vi "Calculo principal.vi"(8 "error in":errorcluster, 11 "Dados SP":T2={"Condutor"={"Pc (N/m)"=0.0, "Mod.Young (N/m²)"=0.0, "Dil.Term.c (m/°C)"=0.0, "Área  (m²)"=0.0, "Tração EDS (N)"=0.0, "Tração Torig(N)"=0.0, "Tração Talta (N)"=0.0}, "Suporte"={"Ps (N/m)"=0.0, "Es (N/m²)"=0.0, "DTc (1/°C)"=0.0, "Área sup (m²)"=0.0, "Tração EDS sup (N)"=0.0, "Tração AT sup (N)"=0.0, "Flecha sup AT (m)"=0.0}, "Projeto"={"Temp. EDS (°C)"=0.0, "Lim.original (°C)"=0.0, "Lim.extend. (°C)"=0.0, "N. cabo/fase"=1.0}, "Vetor de dados"={"Coor.X.esp"=[], "Coor.Y.Esp."=[], "Sub.vao X"=[], "Sub.vao Y"=[], "CoordY.sup"=[], "CoordX.sup"=[]}, "Subvão"={"N. Esp."=0.0, "F.lim (m)"=0.0, "Ext.calc"=0.0, "Ext.definido"=0.0, "Comp.cabo"=0.0, "Ext.55%"=0.0, "Tração sub\nAT (N)"=0.0, "Ext.sel."=0.0, "Flecha lim.\ncalc (m)"=0.0}, "Vão"={"Extensão (m)"=0.0, "Desnivel (m)"=0.0, "Ext.Lim sub (m)"=0.0, "Flecha à 60 °C"=0.0}} {"Projeto"."N. cabo/fase" min=1.0 max=8.0 step=1.0 format="%#_1f"}) -> (0 "error out":errorcluster, 2 "Gráfico":T1(array[cluster]), 3 "Dados SP Out":T2={"Condutor"={"Pc (N/m)"=0.0, "Mod.Young (N/m²)"=0.0, "Dil.Term.c (m/°C)"=0.0, "Área  (m²)"=0.0, "Tração EDS (N)"=0.0, "Tração Torig(N)"=0.0, "Tração Talta (N)"=0.0}, "Suporte"={"Ps (N/m)"=0.0, "Es (N/m²)"=0.0, "DTc (1/°C)"=0.0, "Área sup (m²)"=0.0, "Tração EDS sup (N)"=0.0, "Tração AT sup (N)"=0.0, "Flecha sup AT (m)"=0.0}, "Projeto"={"Temp. EDS (°C)"=0.0, "Lim.original (°C)"=0.0, "Lim.extend. (°C)"=0.0, "N. cabo/fase"=1.0}, "Vetor de dados"={"Coor.X.esp"=[], "Coor.Y.Esp."=[], "Sub.vao X"=[], "Sub.vao Y"=[], "CoordY.sup"=[], "CoordX.sup"=[]}, "Subvão"={"N. Esp."=0.0, "F.lim (m)"=0.0, "Ext.calc"=0.0, "Ext.definido"=0.0, "Comp.cabo"=0.0, "Ext.55%"=0.0, "Tração sub\nAT (N)"=0.0, "Ext.sel."=0.0, "Flecha lim.\ncalc (m)"=0.0}, "Vão"={"Extensão (m)"=0.0, "Desnivel (m)"=0.0, "Ext.Lim sub (m)"=0.0, "Flecha à 60 °C"=0.0}} {"Projeto"."N. cabo/fase" min=1.0 max=8.0 step=1.0 format="%#_1f"})   [LabVIEW 2020]
uses:
  controles/SP data.ctl
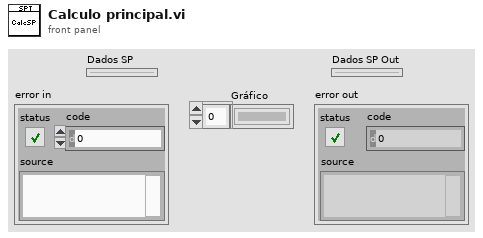
[diagram p1: front panel]
types:
  T1 = cluster{"CoordX.sup":dbl[], "CoordY.sup":dbl[]}[]
  T2 = typedef "SP data.ctl" = cluster{"Condutor":cluster{"Pc (N/m)":dbl, "Mod.Young (N/m²)":dbl, "Dil.Term.c (m/°C)":dbl, "Área  (m²)":dbl, "Tração EDS (N)":dbl, "Tração Torig(N)":dbl, "Tração Talta (N)":dbl}, "Suporte":cluster{"Ps (N/m)":dbl, "Es (N/m²)":dbl, "DTc (1/°C)":dbl, "Área sup (m²)":dbl, "Tração EDS sup (N)":dbl, "Tração AT sup (N)":dbl, "Flecha sup AT (m)":dbl}, "Projeto":cluster{"Temp. EDS (°C)":dbl, "Lim.original (°C)":dbl, "Lim.extend. (°C)":dbl, "N. cabo/fase":dbl}, "Vetor de dados":cluster{"Coor.X.esp":dbl[], "Coor.Y.Esp.":dbl[], "Sub.vao X":dbl[], "Sub.vao Y":dbl[], "CoordY.sup":dbl[], "CoordX.sup":dbl[]}, "Subvão":cluster{"N. Esp.":dbl, "F.lim (m)":dbl, "Ext.calc":dbl, "Ext.definido":dbl, "Comp.cabo":dbl, "Ext.55%":dbl, "Tração sub\nAT (N)":dbl, "Ext.sel.":dbl, "Flecha lim.\ncalc (m)":dbl}, "Vão":cluster{"Extensão (m)":dbl, "Desnivel (m)":dbl, "Ext.Lim sub (m)":dbl, "Flecha à 60 °C":dbl}}
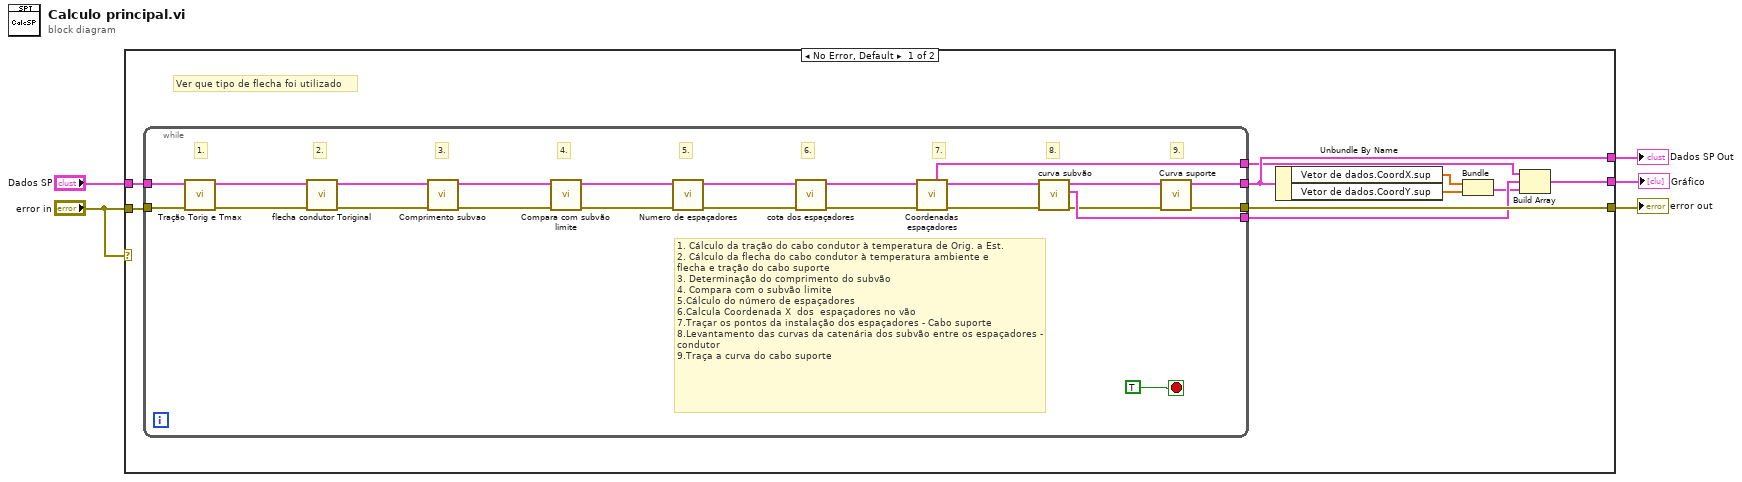
[diagram p0: block diagram]
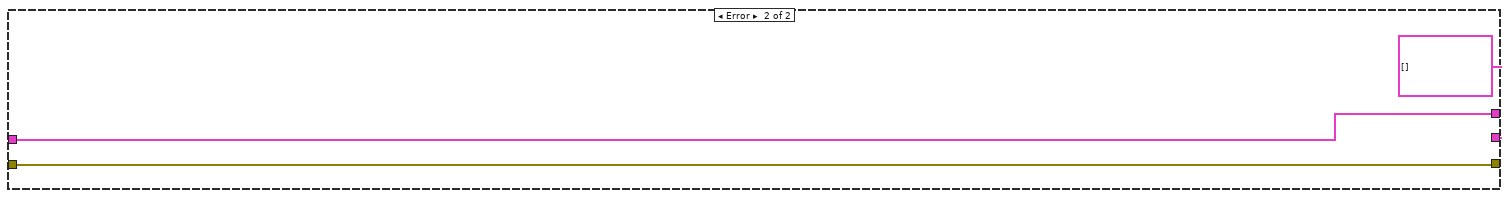
[diagram p2: hidden frame]
diagram:
  n1 = case shown="No Error, Default" "error in" {
    tunnel: "error in" -> [w15 w40]
    tunnel: "Dados SP" -> [w14 w41]
    tunnel: [w13 w40] -> w4
    tunnel: [w12 w41] -> w3
    tunnel: [w6 T1 []] -> w1
    frame No Error {
      # "Ver que tipo de flecha foi utilizado"
      n2 = while {
        tunnel: [w22] -> w11
        tunnel: [w21] -> w10
        tunnel: w14 -> [w37]
        tunnel: [w35] -> w12
        tunnel: w15 -> [w38]
        tunnel: [w36] -> w13
        stop <- TRUE stop-if-true
        # "9."
        # "8."
        # "7."
        # "6."
        # "5."
        # "4."
        # "3."
        # "2."
        # "1."
        # "1. Cálculo da tração do cabo condutor à temperatura de Orig. a Est.\n2. Cálculo da flecha do cabo condutor à temperatura ambiente e\nflecha e tração do cabo suporte\n3. Determinação do comprimento do subvão\n4. Compara com o subvão limite\n5.Cálculo do número de espaçadores\n6.Calcula Coordenada X  dos  espaçadores no vão\n7.Traçar os pontos da instalação dos espaçadores - Cabo suporte\n8.Levantamento das curvas da catenária dos subvão entre os espaçadores - condutor\n9.Traça a curva do cabo suporte"
        n3 = call "Tração Torig e Tmax.vi"("error in (no error)"=w38, "Dados SP"=w37) -> ("error out"=w31:errorcluster, "Dados SP Out"=w32:T2)  [unwired: 8 in]
        n4 = call "flecha condutor Toriginal.vi"("error in (no error)"=w31, "Dados SP"=w32) -> ("error out"=w29:errorcluster, "Dados SP Out"=w30:T2)  [unwired: 8 in]
        n5 = call "Comprimento subvao.vi"("error in (no error)"=w29, "Dados SP"=w30) -> ("error out"=w26:errorcluster, "Dados SP Out"=w28:T2)  [unwired: 8 in]
        n6 = call "Compara com subvão limite.vi"("error in (no error)"=w26, "Dados SP"=w28) -> ("error out"=w25:errorcluster, "Dados SP Out"=w27:T2)  [unwired: 8 in]
        n7 = call "Numero de espaçadores.vi"("error in (no error)"=w25, "Dados SP"=w27) -> ("error out"=w24:errorcluster, "Dados SP Out"=w34:T2)  [unwired: 8 in]
        n8 = call "cota dos espaçadores.vi"("error in"=w24, "Dados SP"=w34) -> ("error out"=w23:errorcluster, "Dados SP Out"=w33:T2)  [unwired: 8 in]
        n9 = call "Coordenadas espaçadores.vi"("error in (no error)"=w23, "Dados SP"=w33) -> ("error out"=w20:errorcluster, "Dados SP Out"=w19:T2, "CoordXY.Esp"=w22:cluster{dbl[], dbl[]})  [unwired: 7 in]
        n10 = call "curva subvão.vi"("error in"=w20, "Dados SP"=w19) -> ("error out"=w17:errorcluster, "Subvão esp."=w21:cluster{dbl[], dbl[]}, "Dados SP Out"=w18:T2)  [unwired: 7 in]
        n11 = call "Curva suporte.vi"("error in (no error)"=w17, "Dados SP"=w18) -> ("error out"=w36:errorcluster, "Dados SP Out"=w35:T2)  [unwired: 8 in]
      }
      n12 = Unbundle By Name(w12) -> ("Vetor de dados.CoordX.sup"=w9:dbl[], "Vetor de dados.CoordY.sup"=w8:dbl[])
      n13 = Bundle("CoordX.sup"=w9, "CoordY.sup"=w8) -> (w7:cluster{"CoordX.sup":dbl[], "CoordY.sup":dbl[]})  [unwired: 1 in]
      n14 = Build Array(w11, w10, w7) -> (w6:T1)
    }
    frame Error {
    }
  }
  "error out" <- w4
  "Dados SP Out" <- w3
  "Gráfico" <- w1
